vi "AlliGator Load SS1 FLI Dataset Prelude.vi"(8 "error in (no error)":errorcluster, 11 "Path in":path) -> (0 "error out":errorcluster, 1 "Metadata":string, 2 "FLI Data File Information":T1, 3 "Path out":path, 4 "Data Description":string)   [LabVIEW 2021, in "AlliGator Files.lvlib"]
doc: "Preliminary steps (optional dialog) in loading a SS1 dataset."
uses:
  AlliGator Files.lvlib
  AlliGator FLI Data File Information.ctl
  Phasor/Phasor Fluorescence Lifetime Parameters v3.ctl
  AlliGator FLI Dataset Type.ctl
  AlliGator Settings List.ctl
  AlliGator Settings.lvlib
  AlliGator HDF5.lvlib
  Phasor/Phasor.lvlib
panel:
  # "see the AlliGator License on the block diagram (Ctrl+E or Window:Show Block Diagram)"
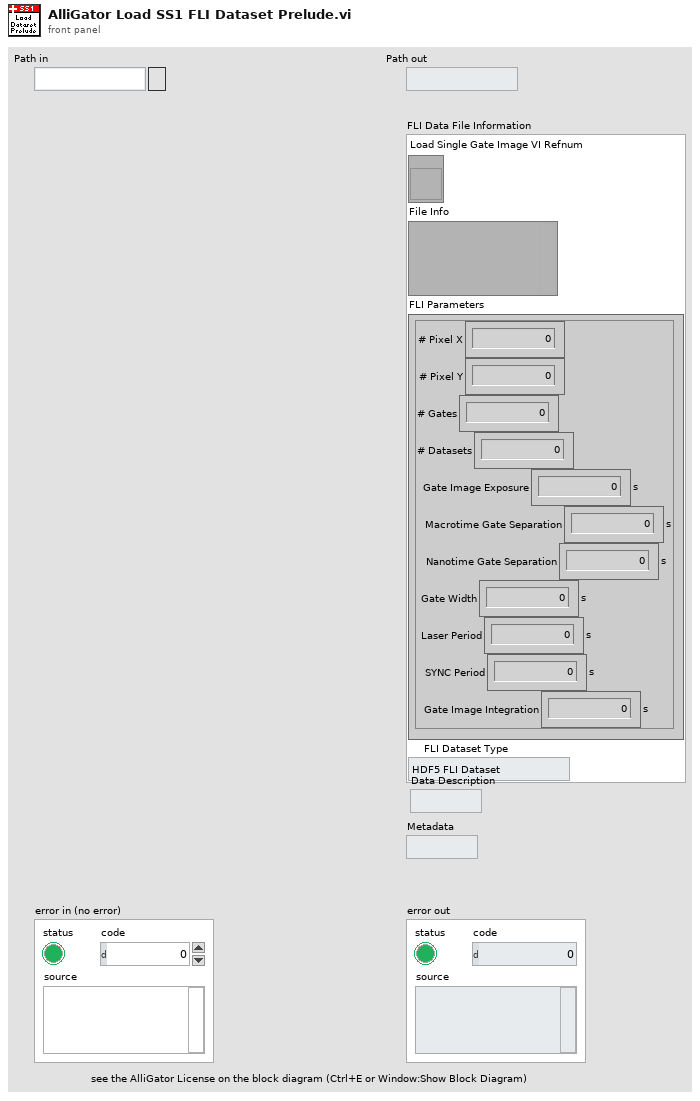
[diagram p1: front panel]
types:
  T1 = typedef "AlliGator HDF5.lvlib/AlliGator FLI Data File Information.ctl" = cluster{"Load Single Gate Image VI Refnum":refnum<vi>, "File Info":variant, "FLI Parameters":T2, "FLI Dataset Type":T3}
  T2 = typedef "Phasor.lvlib/Phasor Fluorescence Lifetime Parameters v3.ctl" = cluster{"# Pixel X":i32, "# Pixel Y":i32, "# Gates":i32, "# Datasets":i32, "Gate Image Exposure":dbl[unit], "Macrotime Gate Separation":dbl[unit], "Nanotime Gate Separation":dbl[unit], "Gate Width":dbl[unit], "Laser Period":dbl[unit], "SYNC Period":dbl[unit], "Gate Image Integration":dbl[unit]}
  T3 = typedef "AlliGator Files.lvlib/AlliGator FLI Dataset Type.ctl" = enum16{"HDF5 FLI Dataset", "Gate Image Folder", ".sdt FLI Dataset (Becker & Hickl)", ".ptu FLI Dataset (PicoQuant)", "SS1 FLI Dataset", "SS2 FLI Dataset", "I/m/phi Dataset", ".bin FLI Dataset (PicoQuant Binned)", ".bin FLI Dataset (Piccolo Binned)"}
  T4 = typedef "AlliGator Settings.lvlib/AlliGator Settings List.ctl" = enum16{"GUI:Visible Settings Tab", "GUI:Last Run Version", "Source Image:Use Image Histogram for Contrast", "Source Image:Low Count Pixels Rejection Options", "Source Image:High Count Pixels Rejection Options", "Source Image:Use Image Brightness", "Source Image:Blend Overlay with Image Background", "Source Image:Use Fixed ROI Diameter", "Source Image:ROI Diameter", "Source Image:ROI Center Color", "Source Image:Peak Threshold", "Source Image:Intensity Threshold", "Source Image:Image Binning Options", "Source Image:Image Smoothing Options", "Source Image:Image Histogram Active", "Source Image:Invert Binary Mask", "Source Image:Hot Pixel Removal", "Source Image:Overlay Analyzed ROI Center", "Source Image:Auto-Adjust Contrast", "Source Image:Histogram Lower Percentile", "Source Image:Histogram Upper Percentile", "Source Image:Save Source Image", "Source Image:Scale Bar Options", "Source Image:Image Resolution (Pixel Size)", "Data Information:Gate Width", "Data Information:Nanotime Gate Separation", "Data Information:Macrotime Gate Separation", "Data Information:Gate Step", "Data Information:# Gates", "Data Information:Gate Image Exposure", "Data Information:Gate Image Integration", "Data Information:Gates to Skip", "Data Information:Gates to Keep", "Data Information:Define Gates to", "Data Information:Channel Name", "Data Information:Available Channel Names", "Data Information:Channel Arithmetic", "Data Information:Background File Subtraction", "Data Information:Background File", "Data Information:Background Scaling Factor", "Data Information:Background Pile-up Correction", "Data Information:Background Pixel Well Capacity", "Data Information:Laser Period", "Data Information:SYNC Period", "Data Information:Pile-up Correction", "Data Information:Pixel Well Capacity", "Data Information:Dataset Scaling Factor", "Fluorescence Decay_Decay Pre-Processing:Reverse Gates", "Fluorescence Decay_Decay Pre-Processing:Verbose Decay Pre-Processing", "Fluorescence Decay_Decay Pre-Processing:Use Decay Pre-Processing", "Fluorescence Decay_Decay Pre-Processing:Background Subtraction", "Fluorescence Decay_Decay Pre-Processing:Background Definition Range", "Fluorescence Decay_Decay Pre-Processing:Baseline Subtraction Method", "Fluorescence Decay_Decay Pre-Processing:Operations Order", "Fluorescence Decay_Decay Pre-Processing:Smoothing Parameter", "Fluorescence Decay_Decay Pre-Processing:Shift Decay", "Fluorescence Decay_Decay Pre-Processing:Decay Shift Parameters", "Fluorescence Decay_Decay Pre-Processing:Fold Decay", "Fluorescence Decay_Decay Pre-Processing:# Folds", "Fluorescence Decay_Decay Pre-Processing:1-Normalize Decay", "Fluorescence Decay_Decay Pre-Processing:[0-1]-Normalize Decay", "Fluorescence Decay_Decay Pre-Processing:Smoothen Decay", "Fluorescence Decay_Decay Pre-Processing:Extrapolate Decay", "Fluorescence Decay_Decay Pre-Processing:Use Periodicity", "Fluorescence Decay_Decay Pre-Processing:Use Cursors", "Fluorescence Decay_Decay Pre-Processing:Tail Fraction", "Fluorescence Decay_Decay Pre-Processing:Head Fraction", "Fluorescence Decay_Decay Pre-Processing:Additional Points", "Fluorescence Decay_Decay Pre-Processing:Straighten Decay", "Fluorescence Decay_Decay Pre-Processing:Constant Background", "Fluorescence Decay_Decay Pre-Processing:Pixel-Normalize Decay", "Fluorescence Decay_Advanced Analysis:Extract IRF instead of Decay", "Fluorescence Decay_Advanced Analysis:IRF Extraction Options", "Fluorescence Decay_Advanced Analysis:IRF Optimization Options", "Fluorescence Decay_Advanced Analysis:Square Pulse Options", "Fluorescence Decay_Advanced Analysis:IRF Order", "Fluorescence Decay_Advanced Analysis:IRF Time Constants", "Fluorescence Decay_Advanced Analysis:Wavelet Analysis Options", "Fluorescence Decay_Advanced Analysis:Average Lifetime Options", "Fluorescence Decay_Fit Options:Fit Options", "Fluorescence Decay_Fit Options:Use Legacy Fitting Approach", "Fluorescence Decay_Fit Options:Use Data Information Laser Period", "Fluorescence Decay_Fit Parameters:Displayed Fit Parameters", "Fluorescence Decay_Fit Parameters:Fit Parameter Constraints", "Fluorescence Decay_Fit Parameters:Export Tabulated Results", "Fluorescence Decay_Fit Parameters:MLE Baseline Offset Type", "Fluorescence Decay_Fit Parameters:MLE Baseline Offset", "Fluorescence Decay_Fit Parameters:Guess Parameter Names", "Fluorescence Decay_Fit Parameters:Guess Parameter Values", "Fluorescence Decay_Fit Parameters:Guess Parameters Options", "Fluorescence Decay_Styles:Show Last Decay Only", "Fluorescence Decay_Styles:Decay Graph Color Array", "Fluorescence Decay:Decay Graph Active", "Fluorescence Decay Statistics:Min Peak Value", "Fluorescence Decay Statistics:Reject Low Decay Peak Pixels", "Fluorescence Decay Statistics:Reject High Decay Peak Pixels", "Fluorescence Decay Statistics:Max Peak Value", "Time Traces:Use File Timestamp", "Time Traces:Time Step", "Time Traces:Use Intensity Correction File", "Time Traces:Intensity Correction File", "Phasor Plot:Phasor Plot Smoothing Options", "Phasor Plot:Phasor Plot Size", "Phasor Plot:Phasor Plot Graphics Options", "Phasor Plot:Cumulative Phasor Plot", "Phasor Plot:Use Phasor Brightness", "Phasor Plot:Blend Overlay with Phasor Background", "Phasor Plot:Save Phasor Plot", "Phasor Plot:Show References", "Phasor Plot:Phasor Ratio Decay Range", "Phasor Plot:Exponential Fading", "Phasor Plot:Phasor Ratio Reference Colors", "Phasor Plot:Reference Radius", "Phasor Plot:Show Color Map Vertices", "Phasor Plot:Phasor Plot Active", "Phasor Plot:Phasor Ratio Color Map Type", "Phasor Plot:Phasor Ratio Color Map", "Phasor Plot:Phasor Ratio Display Range", "Phasor Plot:Selected Image ROI(s)", "Phasor Plot:All Image ROIs", "Phasor Plot:Selected Phasor Plot ROI(s)", "Phasor Plot:All Phasor Plot ROIs", "Phasor Plot:Phasor Ratio Color-Coded Quantity", "Phasor Plot:Store Phasor Harmonics", "Phasor Plot:Draw Reference Segment", "Phasor Plot:User-Defined Quantity", "Phasor Graph:Phasor Frequency", "Phasor Graph:Phasor Ratio Type", "Phasor Graph:Pixel-level Phasor Computation", "Phasor Graph:Save Phasor Graph", "Phasor Graph:Phasor Graph Active", "Phasor Graph:Phasor SDV Options", "Phasor Calibration:Use Backup Calibration if needed", "Phasor Graph:Define Shortest Lifetime as", "Phasor Calibration:Backup Calibration Type", "Phasor Calibration:Calibration Type", "Phasor Calibration:Calibration Lifetime", "Phasor Calibration:Calibration Map Algorithm", "Single-Exponential Phasor Locus (SEPL):Gate Parameters", "Single-Exponential Phasor Locus (SEPL):User-defined Gate", "Single-Exponential Phasor Locus (SEPL):User-defined IRF", "Single-Exponential Phasor Locus (SEPL):Phasor Parameters", "Single-Exponential Phasor Locus (SEPL):Decay & IRF Parameters", "Single-Exponential Phasor Locus (SEPL):Display Parameters", "Lifetime Analysis:Decay Analysis Parameters", "Lifetime Analysis:Lifetime Map Active", "Plugins:Python Settings", "Miscellaneous:Verbose Mode", "Miscellaneous:Beep after Script", "Miscellaneous:Saved Image File Format", "Miscellaneous:Exported Gate Image Settings", "Miscellaneous:Include Loading in Timing", "Miscellaneous:Verbose Settings Mode", "Miscellaneous:Histogram Options", "Miscellaneous:Beep on Error", "Miscellaneous:# Logical Processors Used", "Miscellaneous:ROI Description Max Characters", "Miscellaneous:Verbose Error Mode", "Miscellaneous:Transparent Mask Color"}
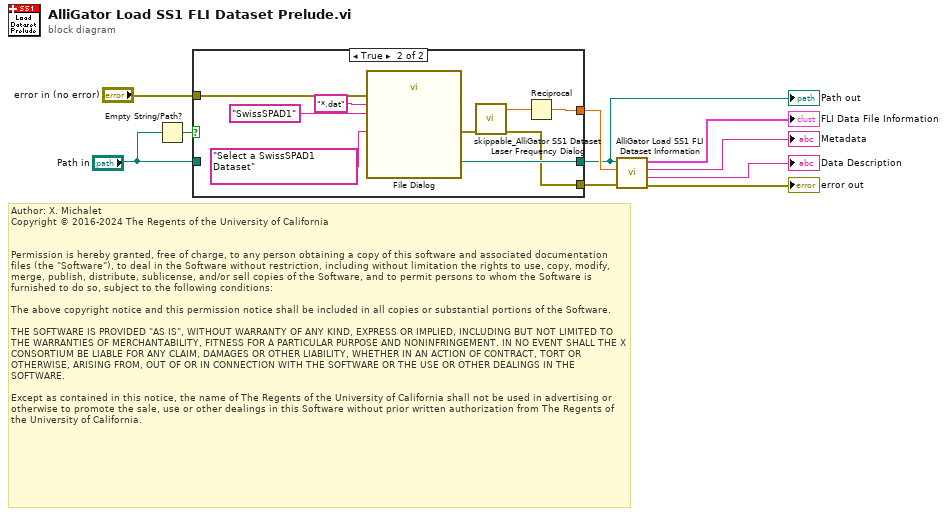
[diagram p0: block diagram]
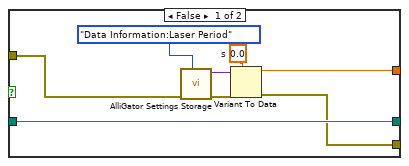
[diagram p2: hidden frame]
diagram:
  # "Author: X. Michalet\nCopyright © 2016-2024 The Regents of the University of California\n \n\nPermission is hereby granted, free of charge, to any person obtaining a copy of this software and associated documentation files (the \"Software\"), to deal in the Software without restriction, including without limitation the rights to use, copy, modify, merge, publish, distribute, sublicense, and/or sell copies of the Software, and to permit persons to whom the Software is furnished to do so, subject to the following conditions:\n\nThe above copyright notice and this permission notice shall be included in all copies or substantial portions of the Software.\n\nTHE SOFTWARE IS PROVIDED \"AS IS\", WITHOUT WARRANTY OF ANY KIND, EXPRESS OR IMPLIED, INCLUDING BUT NOT LIMITED TO THE WARRANTIES OF MERCHANTABILITY, FITNESS FOR A PARTICULAR PURPOSE AND NONINFRINGEMENT. IN NO EVENT SHALL THE X CONSORTIUM BE LIABLE FOR ANY CLAIM, DAMAGES OR OTHER LIABILITY, WHETHER IN AN ACTION OF CONTRACT, TORT OR OTHERWISE, ARISING FROM, OUT OF OR IN CONNECTION WITH THE SOFTWARE OR THE USE OR OTHER DEALINGS IN THE SOFTWARE.\n\nExcept as contained in this notice, the name of The Regents of the University of California shall not be used in advertising or otherwise to promote the sale, use or other dealings in this Software without prior written authorization from The Regents of the University of California."
  n1 = Empty String/Path?(string/path="Path in") -> (empty?=w1:bool)
  n2 = case shown="True" w1 {
    tunnel: "error in (no error)" -> [w12 w27]
    tunnel: [w18 w24] -> w4
    tunnel: [w13 w20] -> w5
    tunnel: "Path in" -> [w18 _]
    tunnel: [w11 w19] -> w10
    frame False {
      w16 = dbl[unit] 0.0  # s
      n3 = call "AlliGator Settings Storage.vi"("AlliGator Settings List"=AlliGator_Settings_List."Data Information:Laser Period", "Error In"=w12) -> ("Error Out"=w14:errorcluster, "Variant Data out"=w17:variant)  [unwired: 8 in]
      n4 = Variant To Data(error in=w14, type=w16, Variant=w17) -> (data=w11:dbl[unit], error out=w13:errorcluster)
    }
    frame True {
      n5 = call "File Dialog"("prompt"="Select a SwissSPAD1 Dataset", "error in"=w27, "pattern (all files)"="*.dat", "pattern label"="SwissSPAD1") -> ("selected path"=w24:path, "error out"=w21:errorcluster)  [unwired: 8 in, 2 out]
      n6 = call "skippable_AlliGator SS1 Dataset Laser Frequency Dialog.vi"("Error In"=w21) -> ("Error Out"=w20:errorcluster, "Laser Frequency"=w22:dbl[unit])  [unwired: 9 in]
      n7 = Reciprocal(x=w22) -> (1/x=w19:dbl[unit])
    }
  }
  "Path out" <- w4
  n8 = call "AlliGator Load SS1 FLI Dataset Information.vi"("error in (no error)"=w5, "Laser Period"=w10, "Image Folder"=w4) -> ("error out"=→"error out":errorcluster, "Data Description"=→"Data Description":string, "Metadata"=→"Metadata":string, "FLI Data File Information"=→"FLI Data File Information":T1)  [unwired: 5 in]
